vi "Open Camera Quick Settings.vi"(8 "error in (no error)":errorcluster, 9 "Open?":bool, 10 "SubPanel Ref":refnum<vi>, 11 "HIJ Vision Camera App in":refnum<class "HIJ Vision Camera App.lvclass">) -> (0 "error out":errorcluster, 3 "HIJ Vision Camera App out":refnum<class "HIJ Vision Camera App.lvclass">)   [LabVIEW 2014, in "HIJ Vision Camera App.lvlib" / "HIJ Vision Camera App.lvclass"]
uses:
  HIJ Vision Camera App.lvclass
  HIJ Vision Camera App.lvclass/HIJ Vision Camera App.ctl
  Camera Actors/IMAQdx Actor/IMAQdx Actor Messages/open camera quick settings Msg/open camera quick settings Msg.lvclass/open camera quick settings Msg.ctl
  <vilib>/ActorFramework/Message Enqueuer/Message Enqueuer.lvclass/Message Enqueuer.ctl
  <vilib>/ActorFramework/Message Enqueuer/Enqueue.vi
  <vilib>/ActorFramework/Message Priority Queue/Priority Enqueue.vi
  Camera Actors/IMAQdx Actor/IMAQdx Actor Messages/open camera quick settings Msg/open camera quick settings Msg.lvclass
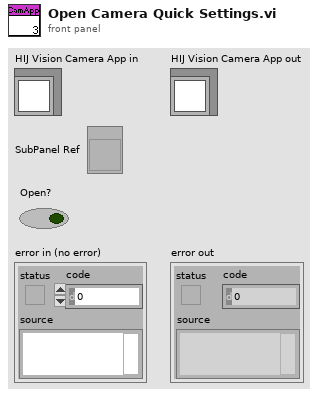
[diagram p1: front panel]
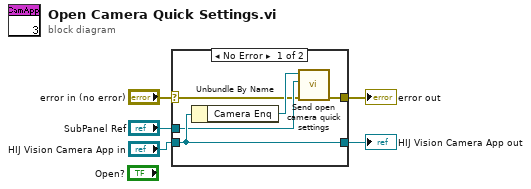
[diagram p0: block diagram]
diagram:
  n1 = case shown="No Error" "error in (no error)" {
    selector: "error in (no error)" -> [w7 w12]
    tunnel: [w6 w12] -> w4
    tunnel: [w10 w11] -> w2
    tunnel: "HIJ Vision Camera App in" -> [w10 w11]
    tunnel: "SubPanel Ref" -> [w8 _]
    frame No Error {
      n2 = Unbundle By Name(w10) -> ("Camera Enq"=w9:refnum<class "Message Enqueuer.lvclass">)
      n3 = call "Send open camera quick settings.vi"("error in (no error)"=w7, "SubPanel Ref"=w8, "Message Enqueuer"=w9) -> ("error out"=w6:errorcluster)  [unwired: 7 in, 1 out]
    }
    frame Error {
    }
  }
  "error out" <- w4
  "HIJ Vision Camera App out" <- w2
